vi "Generate_insert cup locations .vi"() -> ()   [LabVIEW 2019]
panel:
  out "Top":dbl
  out "Middle":dbl
  out "Bottom":dbl
  in  "Lifter reading (mm)":dbl
  in  "Select the cup":T1(radio)
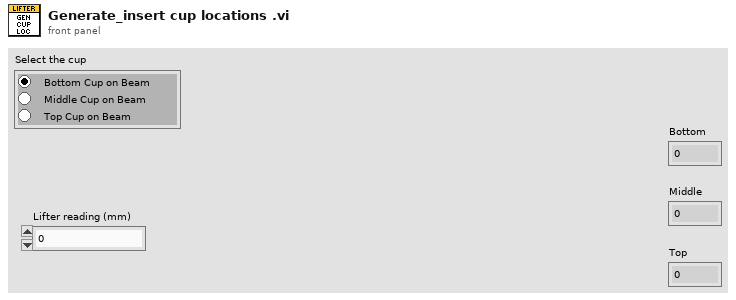
[diagram p1: front panel]
types:
  T1 = enum32{"Bottom Cup on Beam", "Middle Cup on Beam", "Top Cup on Beam"}
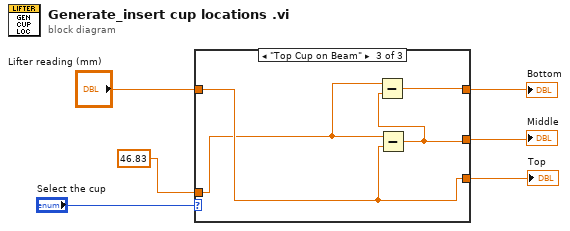
[diagram p0: block diagram]
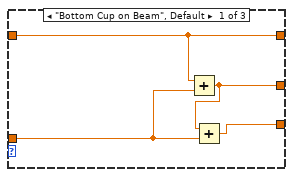
[diagram p2: hidden frame]
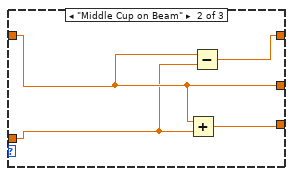
[diagram p3: hidden frame]
diagram:
  n1 = case shown="\"Top Cup on Beam\"" "Select the cup" {
    tunnel: [w10 w14 w17] -> w4
    tunnel: "Lifter reading (mm)" -> [w10 w12 w18]
    tunnel: [w9 w12 w16] -> w3
    tunnel: [w8 w13 w18] -> w2
    tunnel: 46.83 ("y") -> [w7 w11 w15]
    frame "Bottom Cup on Beam", Default {
      n2 = Add(x=w10, y=w7) -> (x+y=w9:dbl)
      n3 = Add(x=w9, y=w7) -> (x+y=w8:dbl)
    }
    frame "Middle Cup on Beam" {
      n4 = Add(x=w12, y=w11) -> (x+y=w13:dbl)
      n5 = Subtract(x=w12, y=w11) -> (x-y=w14:dbl)
    }
    frame "Top Cup on Beam" {
      n6 = Subtract(x=w15, y=w18) -> (x-y=w16:dbl)
      n7 = Subtract(x=w15, y=w16) -> (x-y=w17:dbl)
    }
  }
  "Bottom" <- w4
  "Middle" <- w3
  "Top" <- w2
